vi "_match_enum_from_rangetable.vi"(3 "Smart matching":bool, 4 "Enum string to match":string, 5 "Enums in":T1) -> (0 "Success":bool, 2 "Enum Value out":i32)   [LabVIEW 2020, in "Rohde&Schwarz RTx Oscilloscopes.lvlib" / "rsidr_core.lvlib"]
uses:
  rsidr_core.lvlib
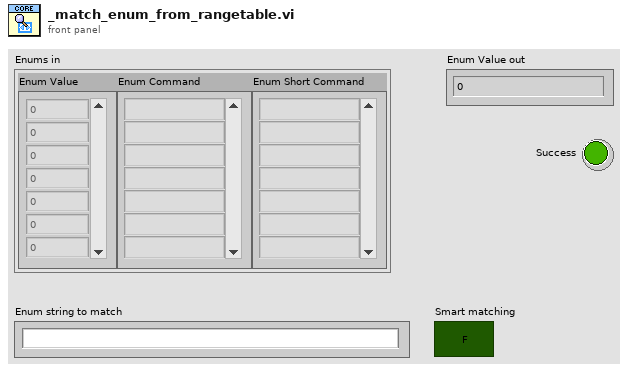
[diagram p1: front panel]
types:
  T1 = cluster{"Enum Value":i32[], "Enum Command":string[], "Enum Short Command":string[]}
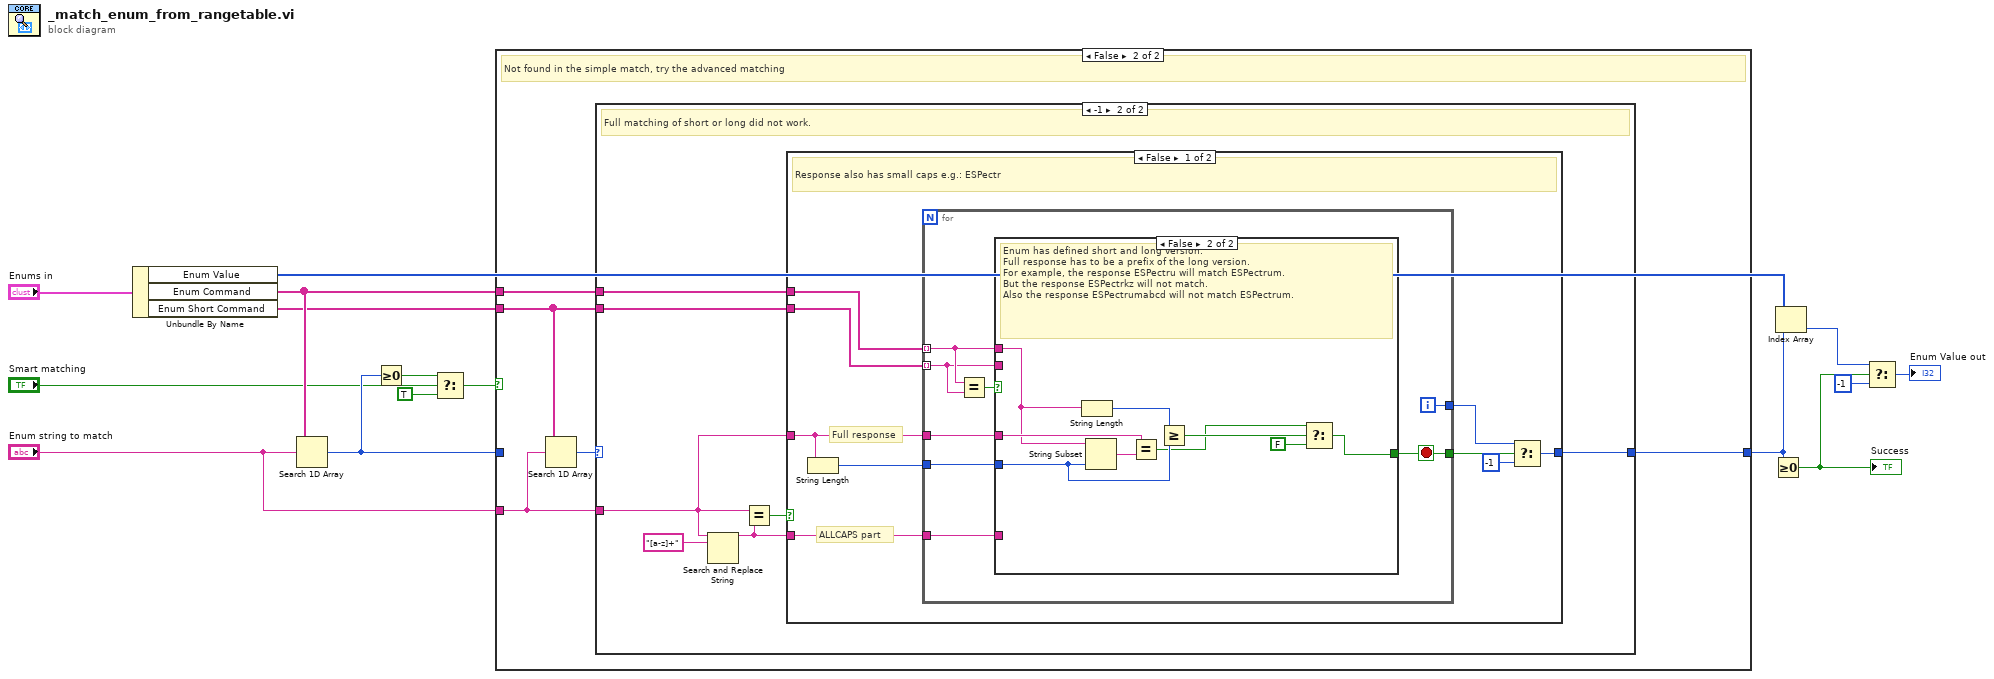
[diagram p0: block diagram]
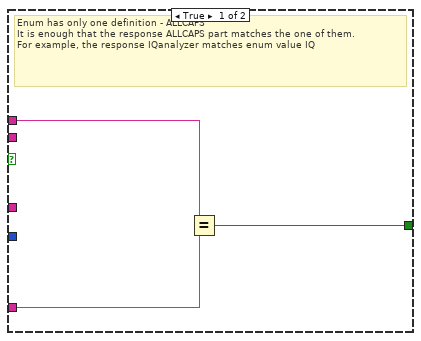
[diagram p4: hidden frame]
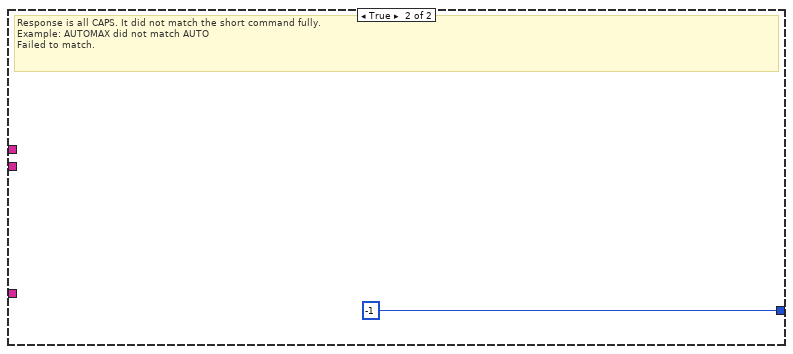
[diagram p5: hidden frame]
diagram:
  n1 = Unbundle By Name("Enums in") -> ("Enum Value"=w10:i32[], "Enum Command"=w14:string[], "Enum Short Command"=w13:string[])
  n2 = Search 1D Array(1D array=w14, element="Enum string to match") -> (index of element=w5:i32)  [unwired: 1 in]
  n3 = Greater Or Equal To 0?(x=w5) -> (x >= 0?=w2:bool)
  n4 = Select(t=w2, s="Smart matching", f=TRUE) -> (s? t:f=w4:bool)
  n5 = case shown="False" w4 {
    tunnel: [w16 w21] -> w6
    tunnel: "Enum string to match" -> [_ w18]
    tunnel: w14 -> [_ w20]
    tunnel: w13 -> [_ w19]
    tunnel: w5 -> [w16 _]
    frame True {
      # "Found in the Enum Command"
    }
    frame False {
      # "Not found in the simple match, try the advanced matching"
      n6 = Search 1D Array(1D array=w19, element=w18) -> (index of element=w17:i32)  [unwired: 1 in]
      n7 = case shown="-1" w17 {
        selector: w17 -> [w22 _]
        tunnel: w18 -> [_ w23]
        tunnel: [w22 w26] -> w21
        tunnel: w19 -> [_ w27]
        tunnel: w20 -> [_ w28]
        frame 0, Default {
          # "Response fully found in the short version (all CAPS)\nFor example, ESP matched command ESPectrum, because its short command is ESP"
        }
        frame -1 {
          # "Full matching of short or long did not work."
          n8 = Search and Replace String(input string=w23, search string="[a-z]+") -> (result string=w25:string)  [unwired: 6 in, 3 out]
          n9 = Equal?(x=w23, y=w25) -> (x = y?=w24:bool)
          n10 = case shown="False" w24 {
            tunnel: w28 -> [w38 _]
            tunnel: w27 -> [w31 _]
            tunnel: [w34 -1 ("f")] -> w26
            tunnel: w25 -> [w30 _]
            tunnel: w23 -> [w37 _]
            frame False {
              # "Full response"
              # "ALLCAPS part"
              # "Response also has small caps e.g.: ESPectr"
              n11 = String Length(string=w37) -> (length=w36:i32)
              n12 = for {
                tunnel: w37 -> [w46]
                tunnel: w38 -> [w42] mode=indexing
                tunnel: w36 -> [w44]
                tunnel: [w45] -> w33
                tunnel: [w43] -> w35
                tunnel: w31 -> [w40] mode=indexing
                tunnel: w30 -> [w39]
                i -> [w45]
                stop <- w43 stop-if-true
                n13 = Equal?(x=w42, y=w40) -> (x = y?=w41:bool)
                n14 = case shown="False" w41 {
                  tunnel: w46 -> [_ w57]
                  tunnel: w42 -> [w48 w56]
                  tunnel: w44 -> [_ w54]
                  tunnel: [w49 w52] -> w43
                  tunnel: w40 -> [_ _]
                  tunnel: w39 -> [w47 _]
                  frame True {
                    # "Enum has only one definition - ALLCAPS\nIt is enough that the response ALLCAPS part matches the one of them.\nFor example, the response IQanalyzer matches enum value IQ"
                    n15 = Equal?(x=w48, y=w47) -> (x = y?=w49:bool)
                  }
                  frame False {
                    # "Enum has defined short and long version.\nFull response has to be a prefix of the long version.\nFor example, the response ESPectru will match ESPectrum.\nBut the response ESPectrkz will not match.\nAlso the response ESPectrumabcd will not match ESPectrum."
                    n16 = String Length(string=w56) -> (length=w55:i32)
                    n17 = String Subset(string=w56, length (rest)=w54) -> (substring=w58:string)  [unwired: 1 in]
                    n18 = Equal?(x=w57, y=w58) -> (x = y?=w51:bool)
                    n19 = Greater Or Equal?(x=w55, y=w54) -> (x >= y?=w53:bool)
                    n20 = Select(t=w51, s=w53, f=FALSE) -> (s? t:f=w52:bool)
                  }
                }
              }
              n21 = Select(t=w33, s=w35, f=-1) -> (s? t:f=w34:i32)
            }
            frame True {
              # "Response is all CAPS. It did not match the short command fully.\nExample: AUTOMAX did not match AUTO\nFailed to match."
            }
          }
        }
      }
    }
  }
  n22 = Greater Or Equal To 0?(x=w6) -> (x >= 0?=w8:bool)
  "Success" <- w8
  n23 = Index Array(array=w10, index=w6) -> (element=w9:i32)
  n24 = Select(t=w9, s=w8, f=-1) -> (s? t:f=→"Enum Value out":i32)
